vi "Pre Launch Init.vi"(11 "Nested in":refnum<class "Home.lvclass">) -> (0 "error out":errorcluster, 3 "Nested out":refnum<class "Home.lvclass">)   [LabVIEW 2020, in "Home.lvlib" / "Home.lvclass"]
doc: "(<B>Filename</B>: Actor Framework.lvlib:Actor.lvclass:Pre Launch Init.vi)\n\nDefines behavior that occurs after the Launch Nested Actor method is invoked but before the actor's Actor Core method begins running.\n\nBy default, this method does nothing. A descendant class may override it to define behavior."
uses:
  Home.lvclass
  Home.lvclass/Home.ctl
  <vilib>/MGI/Panel Manager/Panel Actor/Panel Actor/Panel Actor.lvclass
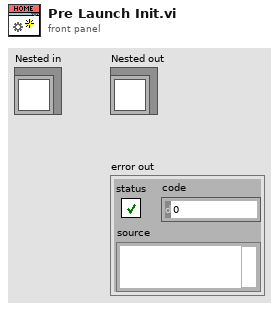
[diagram p1: front panel]
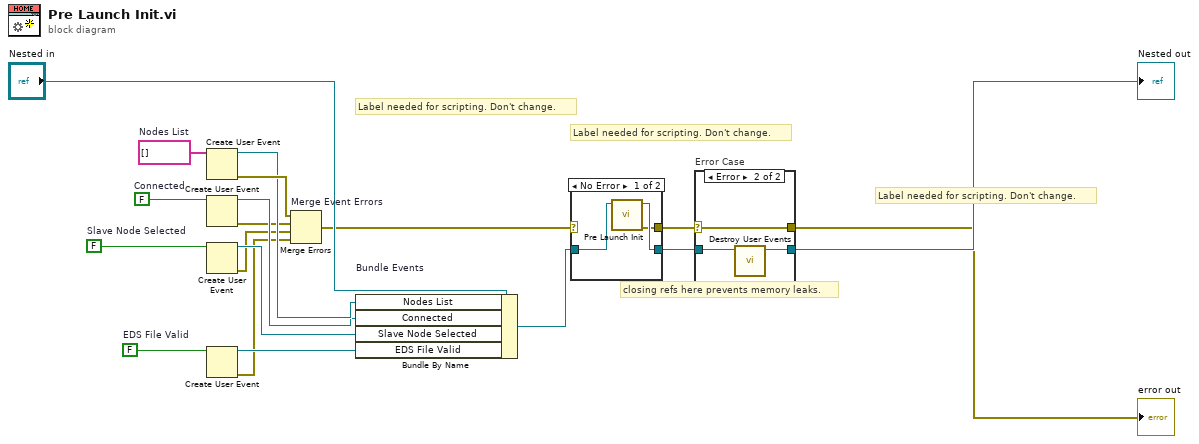
[diagram p0: block diagram]
diagram:
  w3 = FALSE  # EDS File Valid
  w6 = FALSE  # Slave Node Selected
  w9 = FALSE  # Connected
  w11 = string[] []  # Nodes List
  # "Label needed for scripting. Don't change."
  # "Label needed for scripting. Don't change."
  # "Label needed for scripting. Don't change."
  # "closing refs here prevents memory leaks."
  n1 = Create User Event(user event datatype=w11) -> (user event=w10:refnum<user-event>, error out=w18:errorcluster)  [unwired: 1 in]
  n2 = Create User Event(user event datatype=w9) -> (user event=w8:refnum<user-event>, error out=w7:errorcluster)  [unwired: 1 in]
  n3 = Create User Event(user event datatype=w6) -> (user event=w5:refnum<user-event>, error out=w4:errorcluster)  [unwired: 1 in]
  n4 = Create User Event(user event datatype=w3) -> (user event=w2:refnum<user-event>, error out=w1:errorcluster)  [unwired: 1 in]
  n5 = Merge Errors "Merge Event Errors"(w18, w7, w4, w1) -> (w13:errorcluster)
  n6 = Bundle By Name "Bundle Events"(cluster="Nested in", "Nodes List"=w10, "Connected"=w8, "Slave Node Selected"=w5, "EDS File Valid"=w2) -> (w14:refnum<class "Home.lvclass">)
  n7 = case shown="No Error" w13 {
    selector: w13 -> [_ w24]
    tunnel: [w22 w23] -> w15
    tunnel: w14 -> [w21 w23]
    tunnel: [w20 w24] -> w12
    frame No Error {
      n8 = call-parent "Pre Launch Init.vi"("Panel Actor in"=w21) -> ("error out"=w20:errorcluster, "Panel Actor out"=w22:refnum<class "Home.lvclass">)  [unwired: 9 in]
    }
    frame Error {
    }
  }
  n9 = case "Error Case" shown="Error" w12 {
    selector: w12 -> [w25 w29]
    tunnel: w15 -> [w26 w28]
    tunnel: [w26 w27] -> w17
    tunnel: [w25 w29] -> w16
    frame No Error {
    }
    frame Error {
      n10 = call "Destroy User Events.vi"("UI Template in"=w28) -> ("UI Template out"=w27:refnum<class "Home.lvclass">)  [unwired: 10 in]
    }
  }
  "error out" <- w16
  "Nested out" <- w17
